vi "Example.vi"() -> ()   [LabVIEW 2015, in "PPT.lvclass"]
uses:
  PPT.lvclass
  Reusable/Session APIs/File Access/Config Data/Config Data.lvclass
  Instruments/Nicholas/Session/FPGA Serial Session.lvclass
  Instruments/Nicholas/Session/Raw FPGA/FPGA Session.lvclass
  Reusable/Session Log/System Log.lvclass
  Reusable/Session APIs/File Access/Config Data/Config Session.ctl
  Reusable/Session Log/System Log.lvclass/System Log.ctl
  Reusable/Session APIs/File Access/Config Data/Config Data.lvclass/Config Data.ctl
  Instruments/Nicholas/Session/FPGA Serial Session.lvclass/FPGA Serial Session.ctl
  Reusable/Session APIs/Text Communication/Text Device Session.lvclass/Text Device Session.ctl
  Configurable Device/Configurable Device.lvclass/Configurable Device.ctl
  PPT.lvclass/PPT.ctl
  Reusable/Session Log/Accessors/Write Main Path.vi
  Reusable/Session APIs/File Access/Config Data/Accessors/Write Cfg Path.vi
  Instruments/Nicholas/Session/Write fpgaSession.vi
  Reusable/Session APIs/Text Communication/Write hSysLog.vi
  Configurable Device/Write Handle.vi
  Accessors/Write hSession.vi
  Accessors/Write ID.vi
  Reusable/Data/Array Data/Single 1-D/Read Data.vi
  <userlib>/_Session Fwk/Session - Root.lvclass
  Reusable/Data/Array Data/Single 1-D/Single_Array.lvclass
panel:
  out "Data":sgl[](array[numeric])
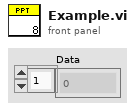
[diagram p1: front panel]
types:
  T1 = typedef "Config Data.lvclass/Config Session.ctl" = refnum<data-value>
  T2 = typedef "Session - Root.lvclass/Session Handle.ctl" = refnum<data-value>
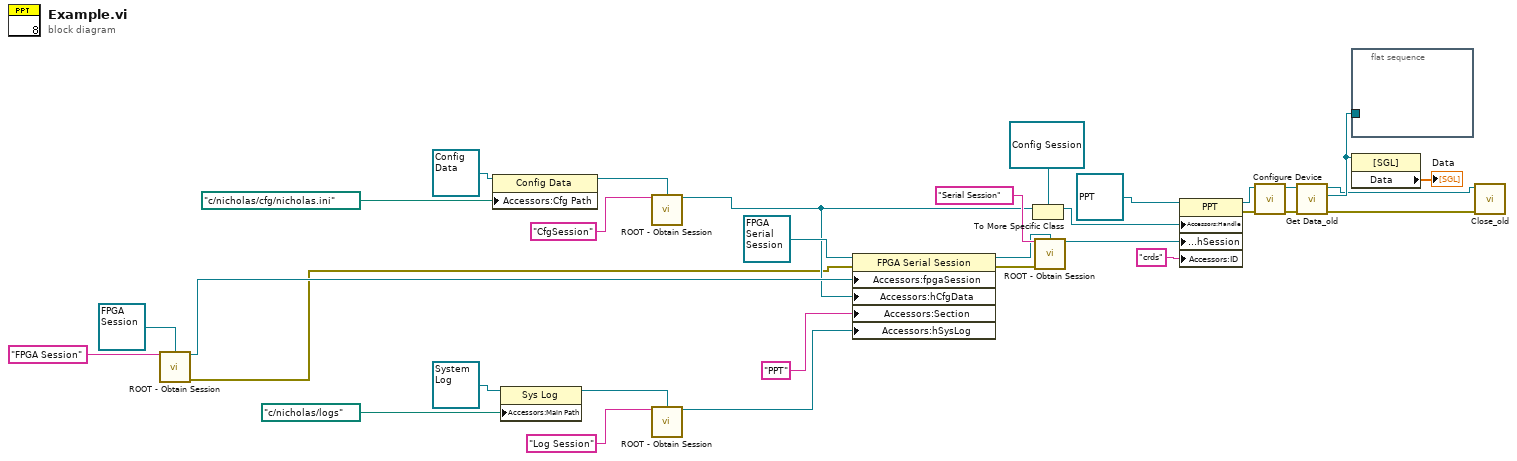
[diagram p0: block diagram]
diagram:
  n1 = call <userlib>:"ROOT - Obtain Session.vi"("Session Name ()"="FPGA Session", "OBJ - Session"=refnum<class "FPGA Session.lvclass"> refnum ("FPGA Session.lvclass")) -> ("Session Handle"=w16:T2, "error out"=w1:errorcluster)  [unwired: 11 in, 1 out]
  n2 = property class="Config Data"(reference=refnum<class "Config Data.lvclass"> refnum ("Config Data"), "Accessors:Cfg Path"=path "c:/nicholas/cfg/nicholas.ini" ("Cfg Path")) -> (reference out=w30:refnum<class "Config Data.lvclass">)  [unwired: 1 in, 1 out]
  n3 = property class="Sys Log"(reference=refnum<class "System Log.lvclass"> refnum ("Sys Log"), "Accessors:Main Path"=path "c:/nicholas/logs" ("Main Path")) -> (reference out=w19:refnum<class "System Log.lvclass">)  [unwired: 1 in, 1 out]
  n4 = call <userlib>:"ROOT - Obtain Session.vi"("Session Name ()"="CfgSession", "OBJ - Session"=w30) -> ("Session Handle"=w15:T2)  [unwired: 11 in, 2 out]
  n5 = call <userlib>:"ROOT - Obtain Session.vi"("Session Name ()"="Log Session", "OBJ - Session"=w19) -> ("Session Handle"=w22:T2)  [unwired: 11 in, 2 out]
  n6 = property class="FPGA Serial Session"(reference=refnum<class "FPGA Serial Session.lvclass"> refnum ("FPGA Serial Session.lvclass"), error in=w1, "Accessors:fpgaSession"=w16, "Accessors:hCfgData"=w15, "Accessors:Section"="PPT" ("Section"), "Accessors:hSysLog"=w22) -> (reference out=w25:refnum<class "FPGA Serial Session.lvclass">, error out=w17:errorcluster)
  n7 = To More Specific Class(target class=T1 refnum ("Handle"), reference=w15) -> (specific class reference=w13:T1)  [unwired: 1 in, 1 out]
  n8 = call <userlib>:"ROOT - Obtain Session.vi"("Session Name ()"="Serial Session", "OBJ - Session"=w25, "error in (no error)"=w17) -> ("Session Handle"=w12:T2)  [unwired: 10 in, 2 out]
  n9 = property class="PPT"(reference=refnum<class "PPT.lvclass"> refnum ("PPT"), "Accessors:Handle"=w13, "Accessors:hSession"=w12, "Accessors:ID"="crds" ("ID")) -> (reference out=w10:refnum<class "PPT.lvclass">, error out=w9:errorcluster)  [unwired: 1 in]
  n10 = call-dynamic "Configure Device.vi"("error in"=w9, "PPT in"=w10) -> ("error out"=w5:errorcluster, "PPT out"=w6:refnum<class "PPT.lvclass">)  [unwired: 8 in]
  n11 = call "Get Data_old.vi"("error in"=w5, "PPT in"=w6) -> ("error out"=w3:errorcluster, "DataOut"=w4:refnum<class "Single_Array.lvclass">, "PPT out"=w2:refnum<class "PPT.lvclass">)  [unwired: 7 in]
  n12 = flat-sequence {
    tunnel: w4 -> [_]
    frame #0 {
    }
  }
  n13 = property class="[SGL]"(reference=w4) -> ("Data"=→"Data":sgl[])  [unwired: 1 in, 2 out]
  n14 = call "Close_old.vi"("error in"=w3, "PPT in"=w2) -> ()  [unwired: 8 in, 2 out]
